vi "数组.vi"() -> ()   [LabVIEW 2017]
panel:
  out "数组 6":dbl[](array[numeric])
  out "数值 2":u16
  out "数值":i32
  in  "数组 5":u16[](array[numeric])
  out "元素 2":string
  out "元素":i32
  out "大小 2":i32[](array[numeric])
  out "大小":i32
  out "数组 4":string[][](array[string])
  in  "数组 3":string[](array[string])
  out "数组 2":dbl[](array[numeric])
  in  "数组":u32[][][](array[numeric])
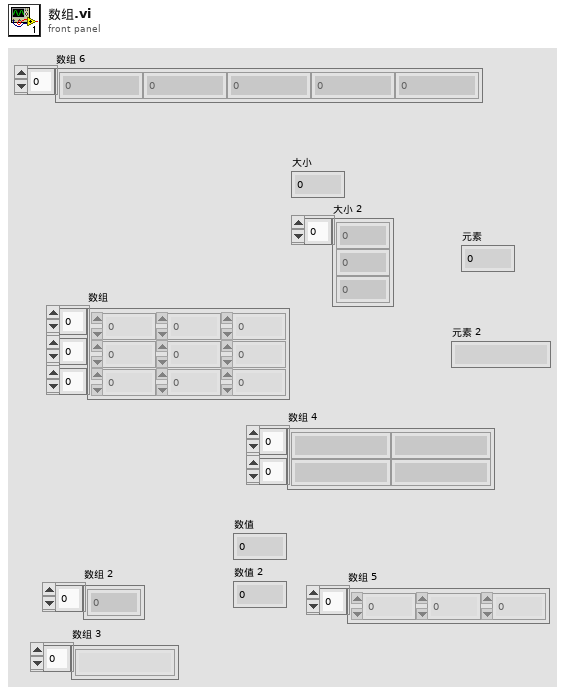
[diagram p1: front panel]
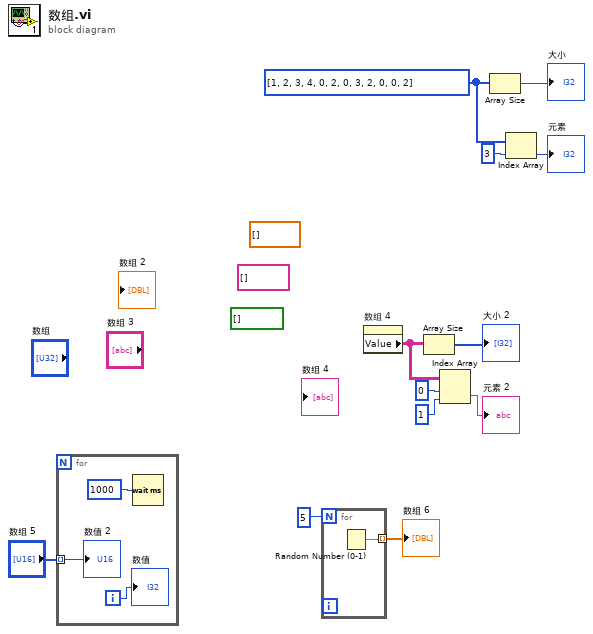
[diagram p0: block diagram]
diagram:
  (unwired) bool[] []
  (unwired) string[] []
  (unwired) dbl[] []
  w10 = i32[] [1, 2, 3, 4, 0, 2, 0, 3, 2, 0, 0, 2]
  n1 = for {
    tunnel: "数组 5" -> [w14] mode=indexing
    i -> [w15]
    n2 = Wait (ms)(milliseconds to wait=u32 1000 ("等待时间（毫秒）")) -> ()  [unwired: 1 out]
    "数值" <- w15
    "数值 2" <- w14
  }
  n3 = for {
    N: 5 -> [_]
    tunnel: [w16] -> w1 mode=indexing
    n4 = Random Number (0-1)() -> (number: 0 to 1=w16:dbl)
  }
  "数组 6" <- w1
  n5 = property on="数组 4" class="Arr (严格)"() -> ("Value"=w7:string[][])  [unwired: 2 in, 2 out]
  n6 = Array Size(array=w7) -> (size(s)=→"大小 2":i32[])
  n7 = Index Array(array=w7, index (row)=0 ("索引 (行)"), index (col)=1 ("禁用的索引 (列)")) -> (element=→"元素 2":string)
  n8 = Array Size(array=w10) -> (size(s)=→"大小":i32)
  n9 = Index Array(array=w10, index=3 ("索引")) -> (element=→"元素":i32)
